vi "static dac defaults.vi"() -> ()   [LabVIEW 2015]
panel:
  out "2ndDAC?":bool=TRUE
  in  "Static DAC scale factor":dbl=1.0
  in  "Dynamic DAC device #":i16=4
  in  "Description DAC":string[](array[string])=["Na Probe Power", "U/D MOT shim", "L/R MOT shim", "F/B MOT shim", "Na Repump Power", "Na Trap Detuning", "Na Trap Power", "Na probe Detuning", "***********************************************", "Rb Trap Detuning (-4.21MHz/Volt) (-4 for MOT)", "QTrap Servo (.5=11A) (5.33*Power voltage(DAC10))", "Power Supply Voltage (1V(control)=6.12V(supply))", "Rb Repump VCO Power out", "IP Quad and Pinch servo ", "IP Bias servo ", "Rb OP/Probe VCO power out", "Rb F = 2 probe detuning"]
  in  "Line 2":i32=15
  in  "Port 2":i32=3
  in  "Static DAQ default volts 2":dbl[](array[numeric])=[-3.5, 0.39, 0.05, -1.1, 0.0, 0.5, -0.6, 0.0] format="%.4f"
  in  "Static DAC device # 2":i16=2
  in  "TTL pulse duration (ms)":dbl=0.001
  in  "Line":i32=14
  in  "Port":i32=3
  in  "Static DAC device #":i16=3
  in  "Static DAQ\ndefault volts":dbl[](array[numeric])=[0.0, 0.18, 0.2, 0.15, -3.0, -0.8, -0.55, 0.0] format="%.4f"
  # "Set up for 2 \"Static\" DAC boards"
  # "TTL trigger for Static DAQ board"
  # "0"
  # "1"
  # "2"
  # "3"
  # "4"
  # "5"
  # "TTL trigger for Static DAQ board"
  # "6"
  # "7"
  # "8"
  # "9"
  # "10"
  # "11"
  # "12"
  # "13"
  # "14"
  # "15"
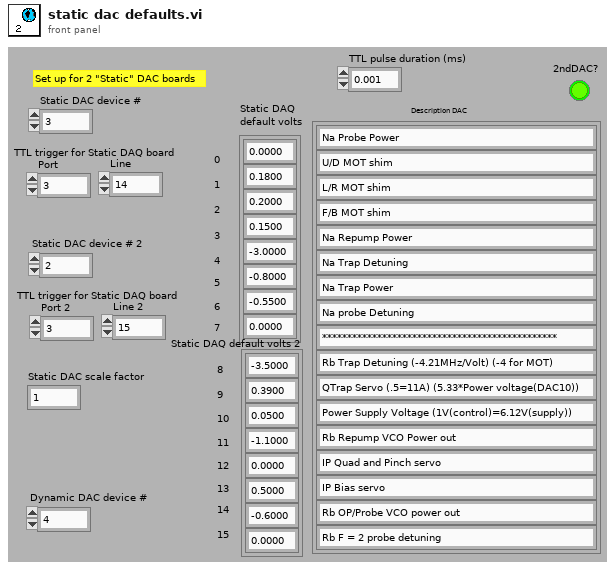
[diagram p1: front panel]
diagram:
